vi "GENser Convert Errors.vi"(8 "error":errorcluster, 9 "Expect \"OK\" (F)":bool, 10 "String in":string, 11 "VISA":refnum<visa-resource-name>="COM1") -> (0 "error out":errorcluster, 3 "VISA out":refnum<visa-resource-name>)   [LabVIEW 2017]
doc: "This vi inputs a string and compares it to all possible Genesys error messages (ex: \"C01\" or \"E04\"). If the response is in the error list, a VISA error number is assigned to it and the error description is passed out the \"error out\" cluster.\n\nIf \"Expect \"OK\"\" is set TRUE, a special error will be passed if the response is not not in the error list and if it is not \"OK\""
panel:
  in  "Error List":T1(array[cluster])=[{"String"="E01", "Code"=-1074001663, "Descr"="<Err>Attemp to set the voltage setting too high. Conflicts with the over-voltage protection."}, {"String"="E02", "Code"=-1074001662, "Descr"="<Err>Attemp to set the voltage setting too low. Conflicts with the under-voltage limit."}, {"String"="E04", "Code"=-1074001660, "Descr"="<Err>Attemp to set the over-voltage protection  too low.  Conflicts with the voltage setting."}, {"String"="E06", "Code"=-1074001658, "Descr"="<Err>Attempt to set the under-voltage limit too high.  Conflicts with the voltage setting."}, {"String"="E07", "Code"=-1074001657, "Descr"="<Err>Attempt to turn the output ON while a fault is keeping the output OFF."}, {"String"="C01", "Code"=-1074001407, "Descr"="<Err>Illegal command or query."}, {"String"="C02", "Code"=-1074001406, "Descr"="<Err>Missing parameter.  Command requires a value but the value is missing."}, {"String"="C03", "Code"=-1074001405, "Descr"="<Err>Illegal parameter.  Command requires a value but value is wrong type."}, {"String"="C04", "Code"=-1074001404, "Descr"="<Err>Checksum error.  Genesys received message with checksum but the checksum did not verify correctly."}, {"String"="C05", "Code"=-1074001403, "Descr"="<Err>Setting out of range.  Attempt to program a setting outside of the model rating."}]
  in  "Qty Elements":i32=10
  # "Convert Errors"
  # "Lambda Genesys \n Serial Port\n  DC Power Supplies"
  # "Match input string to list of\n    Genesys error messages.\nConvert error message to \n    VISA error code."
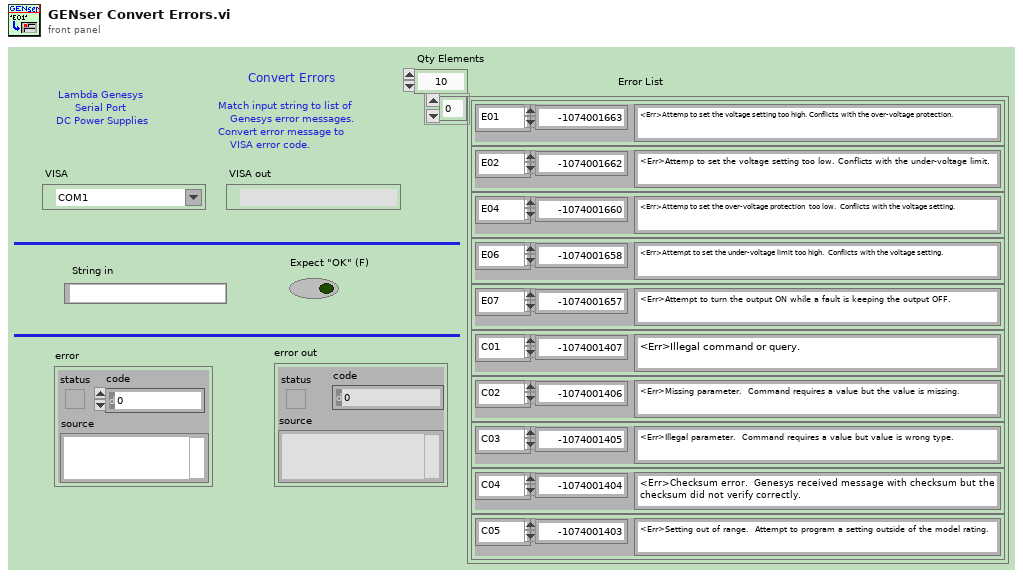
[diagram p1: front panel]
types:
  T1 = cluster{"String":string, "Code":i32, "Descr":string}[]
  T2 = cluster{"String":string, "Code":i32, "Descr":string}
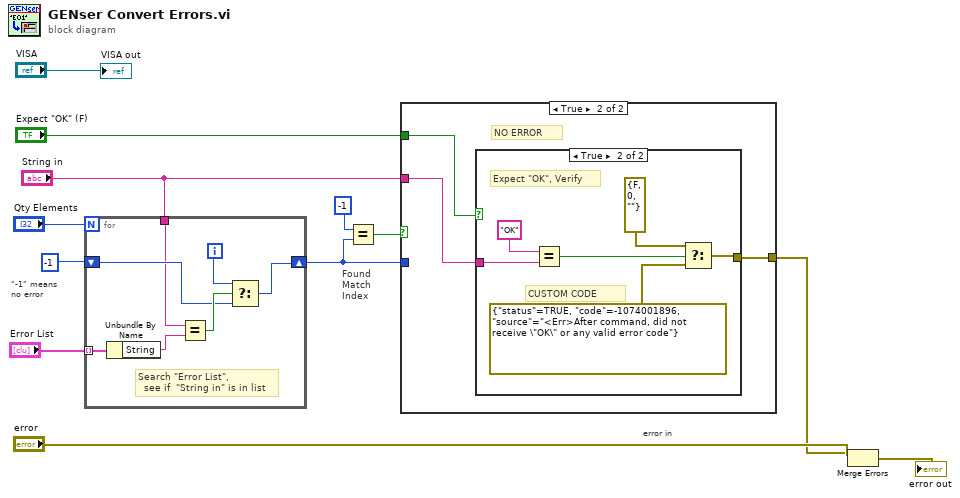
[diagram p0: block diagram]
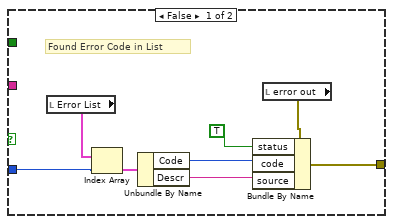
[diagram p2: hidden frame]
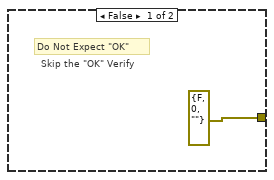
[diagram p3: hidden frame]
diagram:
  # "error in"
  # "Found\nMatch\nIndex"
  # "\"-1\" means\nno error"
  n1 = for {
    N: "Qty Elements" -> [_]
    tunnel: "Error List" -> [w17] mode=indexing
    shift-right: [w14] -> w7
    shift-left: -1 -> [w15]
    tunnel: "String in" -> [w13]
    i -> [w16]
    # "Search \"Error List\", \n  see if  \"String in\" is in list"
    n2 = Unbundle By Name(w17) -> ("String"=w19:string)
    n3 = Equal?(x=w13, y=w19) -> (x = y?=w18:bool)
    n4 = Select(t=w16, s=w18, f=w15) -> (s? t:f=w14:i32)
  }
  n5 = Equal?(x=-1, y=w7) -> (x = y?=w8:bool)
  n6 = case shown="True" w8 {
    tunnel: w7 -> [w25 _]
    tunnel: [w21 w29] -> w4
    tunnel: "String in" -> [_ w30]
    tunnel: "Expect \"OK\" (F)" -> [_ w28]
    frame False {
      # "Found Error Code in List"
      n7 = local read "Error List"() -> (w26:T1)
      n8 = Index Array(array=w26, index=w25) -> (element=w24:T2)
      n9 = Unbundle By Name(w24) -> ("Code"=w23:i32, "Descr"=w20:string)
      n10 = local read "error out"() -> (w27:errorcluster)
      n11 = Bundle By Name(cluster=w27, "status"=TRUE, "code"=w23, "source"=w20) -> (w21:errorcluster)
    }
    frame True {
      # "NO ERROR"
      n12 = case shown="True" w28 {
        tunnel: w30 -> [_ w36]
        tunnel: [errorcluster {"status"=FALSE, "code"=0, "source"=""} ("error") w32] -> w29
        frame False {
          # "Skip the \"OK\" Verify"
          # "Do Not Expect \"OK\""
        }
        frame True {
          # "CUSTOM CODE"
          # "Expect \"OK\", Verify"
          n13 = Equal?(x="OK", y=w36) -> (x = y?=w35:bool)
          n14 = Select(t=errorcluster {"status"=FALSE, "code"=0, "source"=""} ("error"), s=w35, f=errorcluster {"status"=TRUE, "code"=-1074001896, "source"="<Err>After command, did not receive \"OK\" or any valid error code"} ("error")) -> (s? t:f=w32:errorcluster)
        }
      }
    }
  }
  n15 = Merge Errors("error", w4) -> (→"error out":errorcluster)
  "VISA out" <- "VISA"
